vi "Get_USB_Resouce.vi"(8 "error in (no error)":errorcluster) -> (0 "error out":errorcluster, 2 "Get_USB_Resouce":string[](array[string]), 3 "Reference out":refnum<k24>)   [LabVIEW 2017]
doc: "Check usb resource"
uses:
  D:/test/ILSTS/LV_IL_Sample/DLL/InstrumentDLL.dll
  DLL/InstrumentDLL.dll
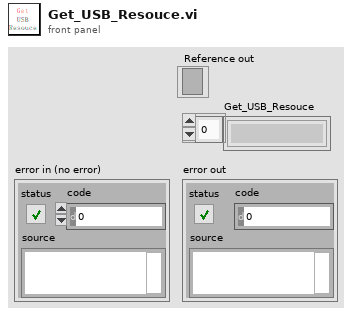
[diagram p1: front panel]
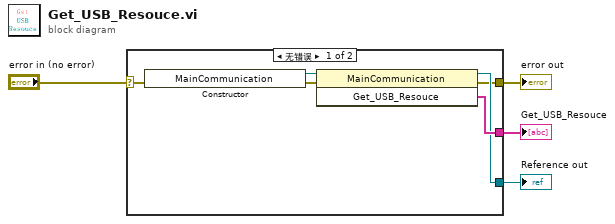
[diagram p0: block diagram]
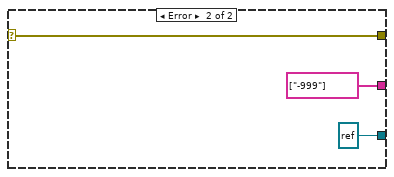
[diagram p2: hidden frame]
diagram:
  n1 = case shown="无错误" "error in (no error)" {
    selector: "error in (no error)" -> [w5 w12]
    tunnel: [w10 string[] ["-999"] ("Get_USB_Resouce")] -> w4
    tunnel: [w7 refnum<k24> refnum ("new reference")] -> w3
    tunnel: [w6 w12] -> w2
    frame No Error {
      n2 = constructor class="MainCommunication"(error in=w5) -> (reference out=w8:refnum<k24>, error out=w9:errorcluster)  [unwired: 2 in, 1 out]
      n3 = invoke on="调用节点" class="MainCommunication" method="Get_USB_Resouce"(reference=w8, error in=w9) -> (reference out=w7:refnum<k24>, error out=w6:errorcluster, "Get_USB_Resouce"=w10:string[])  [unwired: 1 in]
    }
    frame Error {
    }
  }
  "Get_USB_Resouce" <- w4
  "Reference out" <- w3
  "error out" <- w2
